vi "Update Target Tag - PPL Path.vi"(8 "error in (no error)":errorcluster, 10 "exclude dependencies (F)":bool, 11 "Target":refnum<vi>) -> (0 "error out":errorcluster, 2 "Found PPL?":bool, 3 "dup Target":refnum<vi>)   [LabVIEW 2023, in "AFPP Shared.lvlib"]
uses:
  AFPP Shared.lvlib
  Constants.vi
  <vilib>/Utility/error.llb/Error Cluster From Error Code.vi
  <vilib>/ErrorRing/Error Ring.xnode
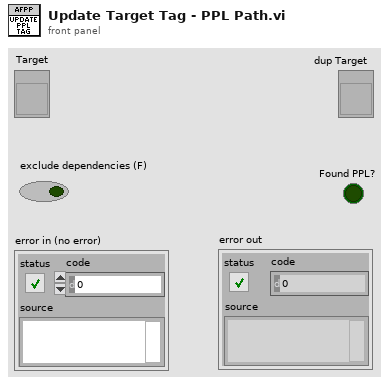
[diagram p1: front panel]
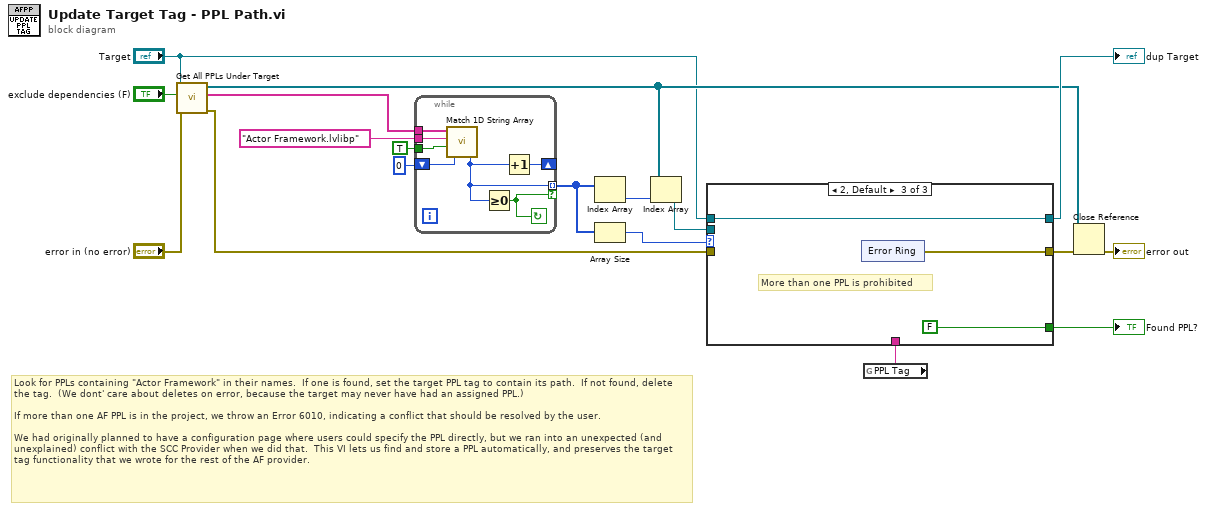
[diagram p0: block diagram]
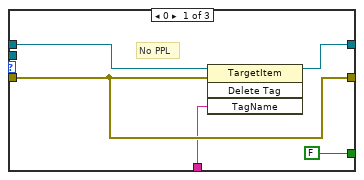
[diagram p2: hidden frame]
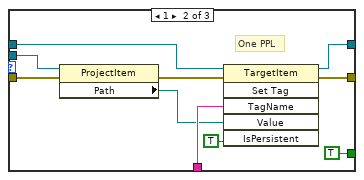
[diagram p3: hidden frame]
diagram:
  # "Look for PPLs containing \"Actor Framework\" in their names.  If one is found, set the target PPL tag to contain its path.  If not found, delete the tag.  (We dont' care about deletes on error, because the target may never have had an assigned PPL.)\n\nIf more than one AF PPL is in the project, we throw an Error 6010, indicating a conflict that should be resolved by the user.\n\nWe had originally planned to have a configuration page where users could specify the PPL directly, but we ran into an unexpected (and unexplained) conflict with the SCC Provider when we did that.  This VI lets us find and store a PPL automatically, and preserves the target tag functionality that we wrote for the rest of the AF provider."
  n1 = call "Get All PPLs Under Target.vi"("error in (no error)"="error in (no error)", "exclude dependencies (F)"="exclude dependencies (F)", "Target"="Target") -> ("error out"=w4:errorcluster, "PPL Names"=w17:string[], "PPLs under target"=w10:refnum<vi>[])  [unwired: 6 in]
  n2 = while {
    tunnel: w17 -> [w25]
    tunnel: "Actor Framework.lvlibp" ("regular expression") -> [w24]
    tunnel: TRUE ("Ignore Case? (false)") -> [w23]
    tunnel: [w20] -> w5 mode=indexing if=w22
    shift-right: [w19] -> _
    shift-left: 0 ("index of element") -> [w21]
    stop <- w22 continue-if-true
    n3 = call <vilib>:"Match 1D String Array.vi"("start index (0)"=w21, "Ignore Case? (false)"=w23, "Pattern"=w24, "Strings"=w25) -> ("index of element"=w20:i32)  [unwired: 1 out]
    n4 = Greater Or Equal To 0?(x=w20) -> (x >= 0?=w22:bool)
    n5 = Increment(x=w20) -> (x+1=w19:i32)
  }
  n6 = Index Array(array=w5) -> (element=w8:i32)  [unwired: 1 in]
  n7 = Array Size(array=w5) -> (size(s)=w2:i32)
  n8 = Index Array(array=w10, index=w8) -> (element=w6:refnum<vi>)
  n9 = global read "Constants.vi" "PPL Tag"() -> (w7:string)
  n10 = case shown="2, Default" w2 {
    tunnel: "Target" -> [w30 w34 w43]
    tunnel: w7 -> [w27 w40 _]
    tunnel: w4 -> [w28 w36 _]
    tunnel: [w28 w38 w42] -> w14
    tunnel: [w29 w37 w43] -> w12
    tunnel: w6 -> [_ w33 _]
    tunnel: [FALSE TRUE FALSE] -> w1
    frame 0 {
      # "No PPL"
      n11 = invoke class="TargetItem" method="Delete Tag"(reference=w30, error in=w28, "TagName"=w27) -> (reference out=w29:refnum<vi>)  [unwired: 1 in, 3 out]
    }
    frame 1 {
      # "One PPL"
      n12 = property class="ProjectItem"(reference=w33, error in=w36) -> (error out=w35:errorcluster, "Path"=w32:path)  [unwired: 1 out]
      n13 = invoke class="TargetItem" method="Set Tag"(reference=w34, error in=w35, "TagName"=w40, "Value"=w32, "IsPersistent"=TRUE ("Is Persistent")) -> (reference out=w37:refnum<vi>, error out=w38:errorcluster)  [unwired: 1 in, 4 out]
    }
    frame 2, Default {
      # "More than one PPL is prohibited"
      n14 = xnode "Error Ring"() -> ("error out"=w42:errorcluster)
    }
  }
  "Found PPL?" <- w1
  "dup Target" <- w12
  n15 = Close Reference(reference=w10, error in (no error)=w14) -> (error out=→"error out":errorcluster)
